vi "SPT Heuristic Solution.vi"(10 "Array":i32[](array[numeric]), 11 "OSSP_Problem in":refnum<class "OSSP_Problem.lvclass">) -> (3 "Scheduled Jobs Order":u16[](array[numeric]))   [LabVIEW 2013, in "GA.lvclass"]
uses:
  GA.lvclass
  OSSP_Problem.lvclass
  GanntChart_Class/Operation to Machine Job Tuple.vi
  GanntChart.lvclass
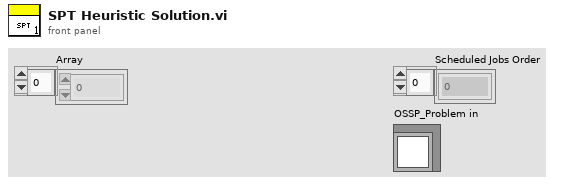
[diagram p1: front panel]
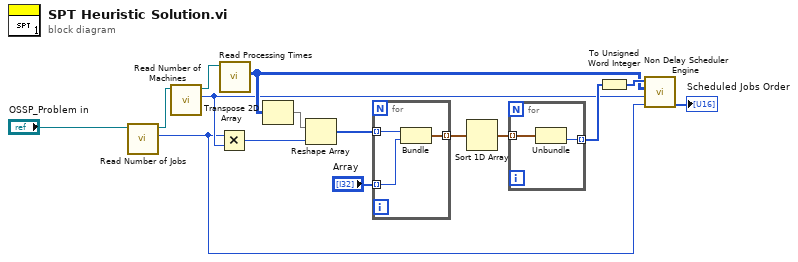
[diagram p0: block diagram]
diagram:
  n1 = call-dynamic "Read Number of Jobs.vi"("OSSP_Problem in"="OSSP_Problem in") -> ("Number of Jobs"=w5:i32, "OSSP_Problem out"=w15:refnum<class "OSSP_Problem.lvclass">)  [unwired: 8 in, 1 out]
  n2 = call-dynamic "Read Number of Machines.vi"("OSSP_Problem in"=w15) -> ("Number of Machines"=w6:i32, "OSSP_Problem out"=w14:refnum<class "OSSP_Problem.lvclass">)  [unwired: 8 in, 1 out]
  n3 = Multiply(x=w5, y=w6) -> (x*y=w12:i32)
  n4 = call-dynamic "Read Processing Times.vi"("OSSP_Problem in"=w14) -> ("Processing Times"=w7:u16[][])  [unwired: 8 in, 2 out]
  n5 = Transpose 2D Array(2D array=w7) -> (transposed array=w13:u16[][])
  n6 = Reshape Array(w13, w12) -> (w11:u16[])
  n7 = for {
    tunnel: w11 -> [w18] mode=indexing
    tunnel: "Array" -> [w17] mode=indexing
    tunnel: [w16] -> w10 mode=indexing
    n8 = Bundle("Numeric"=w18, w17) -> (w16:cluster{"Numeric":u16, i32})  [unwired: 1 in]
  }
  n9 = Sort 1D Array(array=w10) -> (sorted array=w4:cluster{"Numeric":u16, i32}[])
  n10 = for {
    tunnel: w4 -> [w20] mode=indexing
    tunnel: [w19] -> w9 mode=indexing
    n11 = Unbundle(w20) -> (w19:i32)  [unwired: 1 out]
  }
  n12 = To Unsigned Word Integer(number=w9) -> (unsigned 16bit integer=w8:u16[])
  n13 = call "Non Delay Scheduler Engine.vi"("Number of  Jobs"=w5, "Number of Machines"=w6, "Processing Times"=w7, "Schedule"=w8) -> ("Scheduled Jobs Order"=→"Scheduled Jobs Order":u16[])  [unwired: 3 in, 4 out]
